vi "teste-signal-level.vi"() -> ()   [LabVIEW 2014]
uses:
  <vilib>/express/express analysis/Spectral/Block/exnSpectralBlock spectral measurements power poly.vi
  <vilib>/express/express analysis/Spectral/Block/exnSpectralBlock spectral measurements power DDT.vi
  <vilib>/express/express analysis/Spectral/XNode/ExpressSpectralMeasurementsBlockNode.xnode
panel:
  out "Waveform Graph":dynamicdata(graph)
  in  "stop (F)":bool
  out "data":dbl[](graph)
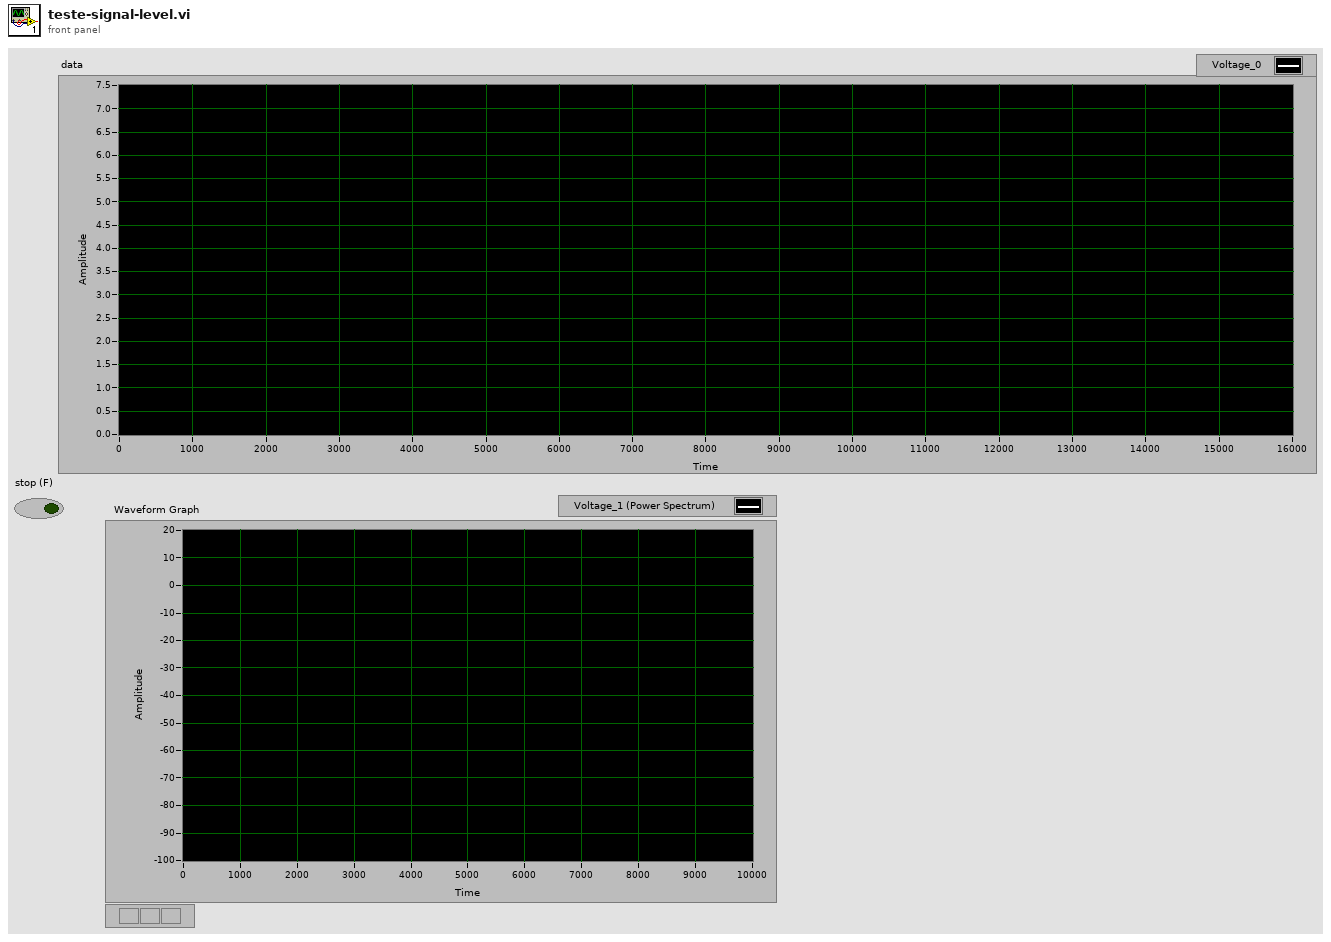
[diagram p1: front panel]
types:
  T1 = cluster{"averaging mode":u16, "weighting mode":u16, "number of averages":u32}
  T2 = cluster{"dB On (F)":bool, "unwrap phase (F)":bool, "convert to degree (F)":bool}
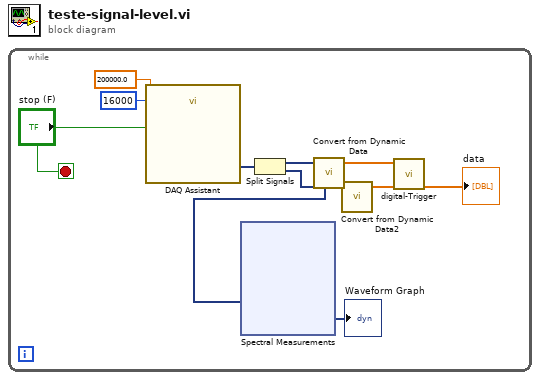
[diagram p0: block diagram]
diagram:
  n1 = while {
    stop <- "stop (F)" stop-if-true
    n2 = call "DAQ Assistant"("rate"=200000.0, "number of samples"=16000, "stop (T)"="stop (F)") -> ("data"=w6:dynamicdata)  [unwired: 14 in, 2 out]
    n3 = Split Signals(w6) -> (w7:dynamicdata, w2:dynamicdata)  [unwired: 2 in]
    n4 = xnode "Spectral Measurements"("Signals"=w2) -> ("Power Spectrum"=→"Waveform Graph":dynamicdata)  [unwired: 1 in, 1 out]
    n5 = call "Convert from Dynamic Data"("Dynamic Data Type"=w7) -> ("Array"=w8:dbl[])  [unwired: 3 in]
    n6 = call "Convert from Dynamic Data2"("Dynamic Data Type"=w2) -> ("Array"=w9:dbl[])  [unwired: 3 in]
    n7 = call "digital-Trigger.vi"("signal in"=w9, "trigger in"=w8) -> ("signal out"=→"data":dbl[])  [unwired: 5 in, 2 out]
  }
